vi "deviceAnalysisTest_StaticOnly.vi"() -> ()   [LabVIEW 2017]
uses:
  <vilib>/addons/InsightCM/MessageBus/Base/KeyValuePairs.ctl
  <vilib>/addons/InsightCM/MessageBus/Base/controls/AlarmRuleEntry.ctl
  <vilib>/addons/InsightCM/Devices/Shared/DataAccessors/controls/channelType_StatusLookup.ctl
  <vilib>/addons/InsightCM/MessageBus/Base/ConfigurableMetric.ctl
  <vilib>/addons/InsightCM/Utilities/ChannelStatus/controls/status.ctl
  <vilib>/addons/InsightCM/Utilities/ChannelStatus/controls/statusState.ctl
  <vilib>/addons/InsightCM/Devices/Shared/ConfigurationParsing/controls/filePaths.ctl
panel:
  out "status changed":bool
  in  "milliseconds to wait":u32=100
  in  "Tab Control":T1(tab)
  in  "Root Directory":path=path "C:/Users/Administrator/Desktop/testDevice files/speedProfile"
  in  "Configuration Files":T2={"AlarmRules"=path "AlarmRules.json", "MetricCfg"=path "MetricConfigs.json", "HierarchyNode"=path "Hierarchy.json", "DeviceModel"=path "DeviceModel.json"}
  in  "Static Values":dbl[](array[numeric])
  out "Waveform Graph":waveform(dbl)[](graph)
  out "FeatureLookup":variant
  in  "stop":bool
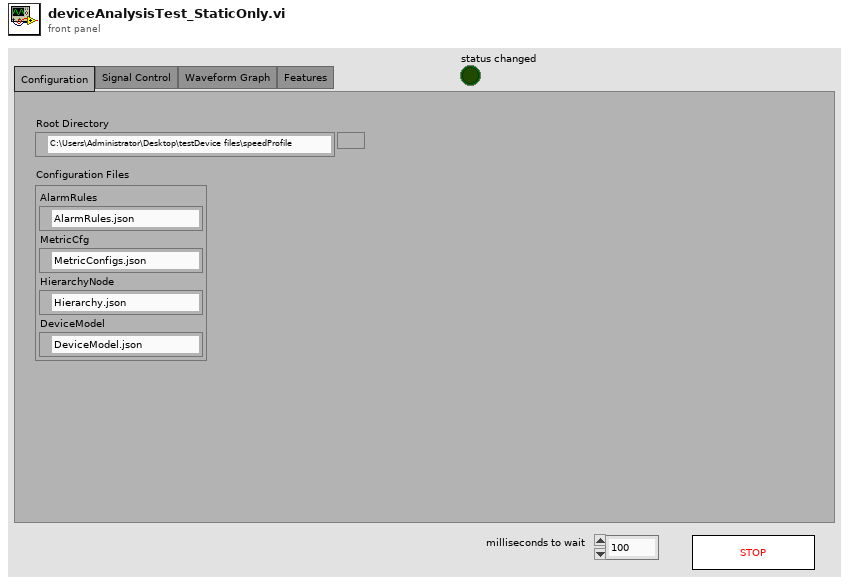
[diagram p1: front panel]
types:
  T1 = enum32{"Configuration", "Signal Control", "Waveform Graph", "Features"}
  T2 = typedef "ConfigurationParsing.lvlib/filePaths.ctl" = cluster{"AlarmRules":path, "MetricCfg":path, "HierarchyNode":path, "DeviceModel":path}
  T3 = typedef "ChannelStatus.lvlib/statusState.ctl" = cluster{"channelAlias":string, "current":T4, "previous":T4, "changed":bool}
  T4 = typedef "ChannelStatus.lvlib/status.ctl" = enum16{"init", "ok", "open", "short", "outOfRange"}
  T5 = typedef "ConfigurableMetric.ctl" = cluster{"Id":i32, "MetricType":string, "Name":string, "Locked":bool, "Properties":T6}
  T6 = typedef "KeyValuePairs.ctl" = cluster{"Key":string, "Value":string}[]
  T7 = typedef "AlarmRuleEntry.ctl" = cluster{"Id":i32, "State":string, "Path":string, "Message":string, "DeviceOnly":bool, "Configuration":cluster{"Condition":string, "SetPoint":string, "Type":string, "Hysteresis":dbl, "OnDelaySeconds":dbl, "OffDelaySeconds":dbl}, "Severity":i32}
  T8 = typedef "ConfigurationParsing.lvlib/DeviceConfigData.ctl" = cluster{"Device Info":T9, "AcquisitionProperties":variant, "Channels":variant[], "StreamingProperties":variant, "DeviceSystemProperties":variant}
  T9 = typedef "ConfigurationParsing.lvlib/deviceInfo.ctl" = cluster{"Config Version":string, "DeviceID":string}
  T10 = typedef "DeviceModel.ctl" = cluster{"AssetModel":T11, "SoftwareModel":T12}
  T11 = typedef "AssetModel.ctl" = cluster{"Id":i32, "PhysicalName":string, "LogicalName":string, "PluginCodename":string, "FirmwareInfo":string, "HardwareConfig":string, "SoftwareConfigId":i32, "HierarchyNodeId":i32}
  T12 = typedef "SoftwareModel.ctl" = cluster{"Id":i32, "DeviceAssetModelId":i32, "Version":string, "Config":string, "DeviceProperties":T6, "Channels":T13[]}
  T13 = typedef "BlueRidgeChannel.ctl" = cluster{"Id":i32, "ChannelId":string, "Name":string, "ChannelCategory":string, "ChannelType":string, "ChannelTypeList":string, "HierarchyNodeId":i32, "Enabled":bool, "Properties":T6, "MetricConfigurations":T14[]}
  T14 = typedef "MetricConfiguration.ctl" = cluster{"Id":i32, "ChannelCategory":string, "MeasurementType":string, "Metrics":T15[]}
  T15 = typedef "MetricInstance.ctl" = cluster{"Id":i32, "Codename":string, "DisplayName":string, "Unit":string, "PublishToHistorian":bool, "Unscaled":bool, "Locked":bool, "TagPath":string, "Properties":T6}
  T16 = cluster{"AlarmRules":variant, "MetricCfg":variant, "HierarchyNode":variant, "DeviceConfig":T8, "DeviceModel":T10}
  T17 = typedef "AnalysisDevice.ctl" = cluster{"Device Id":string, "Dynamic Channels":T18[], "Static Channels":T26[]}
  T18 = typedef "AnalysisDynamicChannel.ctl" = cluster{"ChannelName":string, "Sensor Type":T19, "Conversion Op":T20, "Features":T21[], "Data":waveform(sgl), "Speed":sgl, "SP Index":i32, "Properties":variant, "Data Valid":bool, "Calc Measurement Type":T25}
  T19 = typedef "AnalysisSensorType.ctl" = enum16{"Accelerometer", "Velocity", "Displacement", "Tachometer", "Tempertature ", "dynamicVoltage", "Voltage", "Current", "Microphone", "Resistance", "Digital Input", "<Unknown>"}
  T20 = typedef "AnalysisConversionOp.ctl" = enum16{"none", "singleInt", "doubleInt", "singleDiff", "doubleDiff"}
  T21 = typedef "AnalysisFeature.ctl" = cluster{"Type":i32, "Code Name":string, "Unit":string, "Display Name":string, "Value":sgl, "Start":dbl, "Stop":dbl, "Band Domain":T22, "Band Calc":T23, "Amplitude Scale":T24, "Tag Path":string}
  T22 = typedef "AnalysisBandDomain.ctl" = enum16{"Frequency", "CPM", "Orders"}
  T23 = typedef "AnalysisBandCalculation.ctl" = enum16{"Total", "Max", "Phase"}
  T24 = typedef "AnalysisBandAmplitudeScale.ctl" = enum16{"rms", "peak", "pk-pk", "phase", "<none>"}
  T25 = typedef "AnalysisCalculatedMeasurementType.ctl" = enum16{"acceleration", "velocity", "displacement", "tachometer", "speed", "temperature", "voltage", "current", "resistance", "digitalInput", "<Unknown>"}
  T26 = typedef "AnalysisStaticChannel.ctl" = cluster{"ChannelName":string, "Sensor Type":T19, "Features":T21[], "Properties":variant, "Data Valid":bool, "Calc Measurement Type":T25, "Acquisition Timestamp":timestamp}
  T27 = typedef "AnalysisState.ctl" = cluster{"Properties":cluster{"File Properties":variant, "Static Properties":variant, "Waveform Properties":variant}, "Properties Initialized?":bool, "Device":T17, "Speed Profiles":T28[]}
  T28 = typedef "AnalysisSpeedProfile.ctl" = cluster{"t0":dbl, "pulse positions":sgl[], "speed":dbl}
  T29 = typedef "AnalysisBOP.lvlib/AnalysisGroups.ctl" = cluster{"StaticChannels":T30[], "TachVibrationGroups":T32[]}
  T30 = typedef "AnalysisBOP.lvlib/GeneralStaticChanAnalysisCfg.ctl" = cluster{"Wfm Index":i32, "ChannelName":string, "ChannelID":string, "bounds":T31, "TagPath":string, "Triggerable":bool}
  T31 = typedef "ChannelStatus.lvlib/outOfRangeBounds.ctl" = cluster{"maximum":dbl, "minimum":dbl}
  T32 = typedef "AnalysisBOP.lvlib/TachVibrationGroupCfg.ctl" = cluster{"TachometerChanAnalysisConfig":T33, "AnalysisChannels":T34[]}
  T33 = typedef "AnalysisBOP.lvlib/TachometerChanAnalysisCfg.ctl" = cluster{"Wfm Index":i32, "ChannelName":string, "ChannelID":string, "PulsesPerRevolution":sgl, "TachometerThreshold":sgl, "TachometerSlope":string, "TachometerHysteresis":sgl, "sampleRate":dbl, "tachometerType":string, "Analysis Wfm Index":i32}
  T34 = typedef "AnalysisBOP.lvlib/VibrationChanAnalysisCfg.ctl" = cluster{"Wfm Index":i32, "ChannelName":string, "ChannelID":string, "speedRatio":dbl, "MeasurementType":string}
  T35 = typedef "channelType_StatusLookup.ctl" = enum16{"Static", "Dynamic"}
  T36 = typedef "wfmSGL_DVR.ctl" = refnum<data-value>
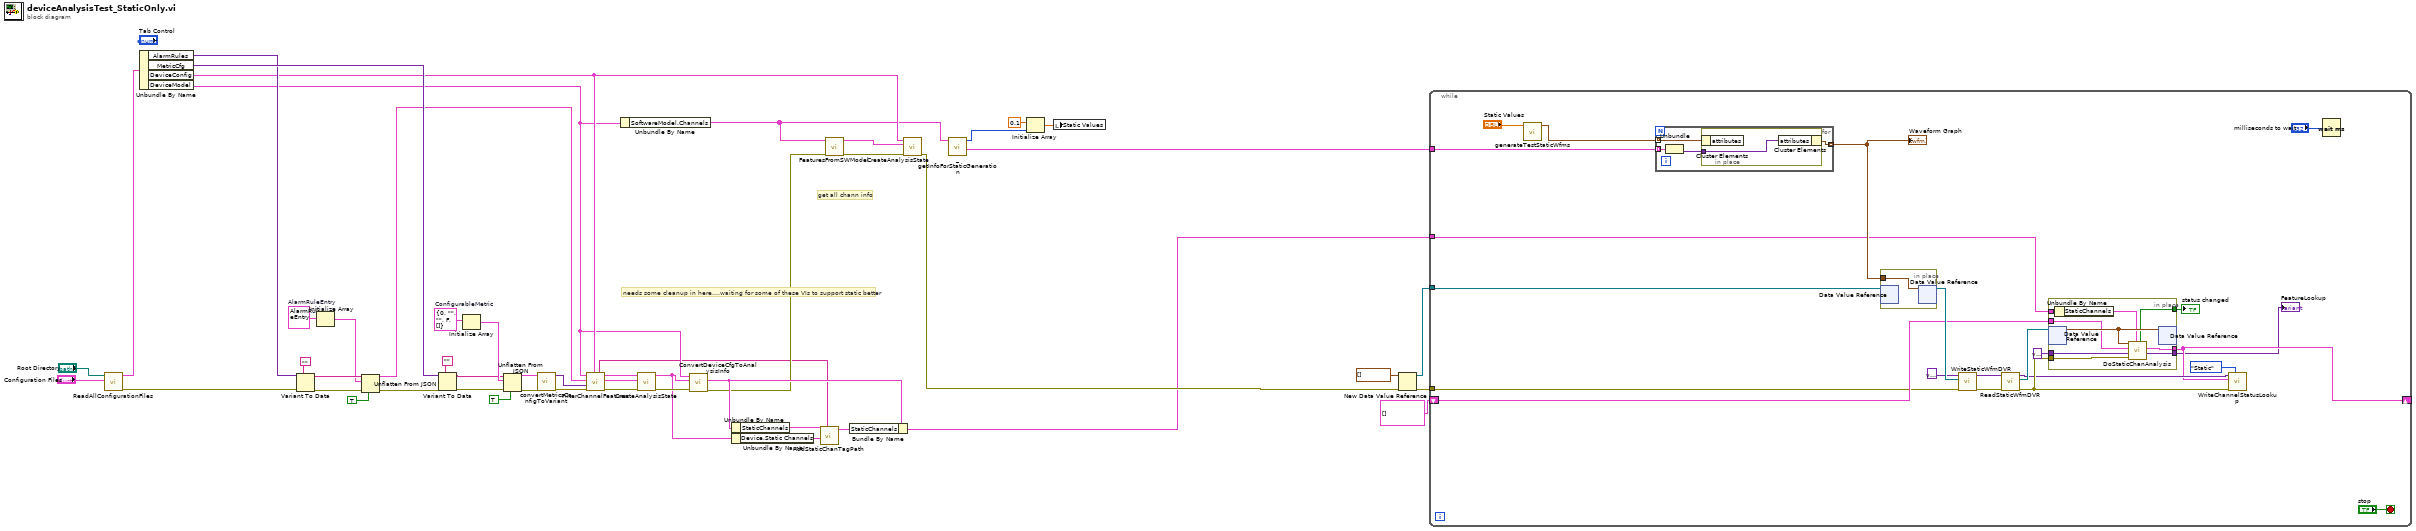
[diagram p0: block diagram]
diagram:
  w22 = T5 {"Id"=0, "MetricType"="", "Name"="", "Locked"=FALSE, "Properties"=[]}  # ConfigurableMetric
  w34 = T7 {"Id"=0, "State"="", "Path"="", "Message"="", "DeviceOnly"=FALSE, "Configuration"={"Condition"="", "SetPoint"="", "Type"="", "Hysteresis"=0.0, "OnDelaySeconds"=0.0, "OffDelaySeconds"=0.0}, "Severity"=0}  # AlarmRuleEntry
  # "needs some cleanup in here....waiting for some of these VIs to support static better"
  # "get all chann info"
  n1 = call <vilib>:"ReadAllConfigurationFiles.vi"("Configuration Files"="Configuration Files", "Root Directory"="Root Directory") -> ("error out"=w7:errorcluster, "Configuration"=w46:T16)  [unwired: 6 in, 2 out]
  n2 = Unbundle By Name(w46) -> ("AlarmRules"=w31:variant, "MetricCfg"=w40:variant, "DeviceConfig"=w20:T8, "DeviceModel"=w3:T10)
  n3 = Variant To Data(error in=w7, type="", Variant=w31) -> (data=w35:string, error out=w37:errorcluster)
  n4 = Initialize Array(w34) -> (w33:T7[])  [unwired: 1 in]
  n5 = Unflatten From JSON(JSON string=w35, type and defaults=w33, default null elements? (F)=TRUE, error in (no error)=w37) -> (value=w23:T7[], error out=w32:errorcluster)  [unwired: 3 in]
  n6 = Variant To Data(error in=w32, type="", Variant=w40) -> (data=w41:string, error out=w44:errorcluster)
  n7 = Initialize Array(w22) -> (w42:T5[])  [unwired: 1 in]
  n8 = Unflatten From JSON(JSON string=w41, type and defaults=w42, default null elements? (F)=TRUE, error in (no error)=w44) -> (value=w39:T5[], error out=w30:errorcluster)  [unwired: 3 in]
  n9 = call <vilib>:"convertMetricsConfigToVariant.vi"("error in (no error)"=w30, "MetricInstanceConfigs"=w39) -> ("error out"=w47:errorcluster, "metricInstanceConfig"=w24:variant)  [unwired: 8 in]
  n10 = call <vilib>:"FilterChannelFeatures.vi"("DeviceConfig"=w20, "error in (no error)"=w47, "Metric Lookup"=w24, "AlarmRules"=w23, "DeviceModel"=w3) -> ("error out"=w50:errorcluster, "Device"=w48:T17, "DeviceConfig Out"=w49:T8, "trigger list"=w2:string[])  [unwired: 3 in]
  n11 = Unbundle By Name(w3) -> ("SoftwareModel.Channels"=w13:T13[])
  n12 = call <vilib>:"CreateAnalysisState.vi"("error in (no error)"=w50, "Device"=w48, "DeviceConfig"=w49) -> ("error out"=w6:errorcluster, "Analysis State"=w4:T27)  [unwired: 7 in]
  n13 = call <vilib>:"ConvertDeviceCfgToAnalysisInfo.vi"("error in (no error)"=w6, "Analysis State"=w4, "DeviceModel"=w3) -> ("error out"=w5:errorcluster, "AnalysisGroups"=w9:T29)  [unwired: 5 in, 2 out]
  n14 = Unbundle By Name(w9) -> ("StaticChannels"=w11:T30[])
  n15 = Unbundle By Name(w4) -> ("Device.Static Channels"=w12:T26[])
  n16 = call <vilib>:"AddStaticChanTagPath.vi"("trigger list"=w2, "Device.Static Channels"=w12, "StaticChannels"=w11) -> ("StaticChannels out"=w10:T30[])  [unwired: 8 in]
  n17 = call <vilib>:"FeaturesFromSWModel.vi"("error in (no error)"=w5, "Channels"=w13) -> ("error out"=w15:errorcluster, "Device"=w14:T17)  [unwired: 8 in]
  n18 = Bundle By Name(cluster=w9, "StaticChannels"=w10) -> (w8:T29)
  n19 = call <vilib>:"CreateAnalysisState.vi"("error in (no error)"=w15, "Device"=w14, "DeviceConfig"=w20) -> ("error out"=w21:errorcluster)  [unwired: 7 in, 1 out]
  n20 = call <vilib>:"_getInfoForStaticGeneration.vi"("Channels"=w13) -> ("wfm info"=w19:cluster{i32, "variant":variant}[], "number of channels"=w18:i32)  [unwired: 9 in]
  n21 = Initialize Array(0.1 ("element"), w18) -> (w16:dbl[])
  n22 = local write "Static Values"(w16) -> ()
  n23 = New Data Value Reference(data value=waveform(sgl)[] [] ("wfmData"), error in=w21) -> (data value reference=w26:refnum<data-value>, error out=w27:errorcluster)
  n24 = while {
    tunnel: w27 -> [w53]
    tunnel: w8 -> [w54]
    shift-right: [w59] -> _
    shift-left: T3[] [] ("channel status") -> [w57]
    tunnel: w26 -> [w72]
    tunnel: w19 -> [w68]
    stop <- "stop" stop-if-true
    n25 = call <vilib>:"generateTestStaticWfms.vi"("Static Values"="Static Values") -> ("waveforms"=w52:waveform(dbl)[])  [unwired: 10 in]
    n26 = for {
      tunnel: w52 -> [w84] mode=indexing
      tunnel: w68 -> [w85] mode=indexing
      tunnel: [w83] -> w67 mode=indexing
      n27 = Unbundle(w85) -> ("variant"=w82:variant)  [unwired: 1 out]
      n28 = in-place {
        in-place-border: w82 -> [w86]
        n29 = in-place-cluster #1(w84) -> ()  [unwired: 1 out]
        n30 = in-place-cluster #1("attributes"=w86) -> (w83:waveform(dbl))
      }
    }
    "Waveform Graph" <- w67
    n31 = in-place {
      in-place-border: w67 -> [w87]
      n32 = in-place-dvr #2(w72) -> ()  [unwired: 2 out]
      n33 = in-place-dvr #2(w87) -> (w71:refnum<data-value>)  [unwired: 1 out]
    }
    n34 = call <vilib>:"WriteStaticWfmDVR.vi"("error in (no error)"=w53, "staticWfmDVR"=w71, "variant"=variant) -> ("error out"=w61:errorcluster, "variant"=w60:variant)  [unwired: 7 in]
    n35 = call <vilib>:"ReadStaticWfmDVR.vi"("error in (no error)"=w61, "variant"=w60) -> ("error out"=w63:errorcluster, "staticWfmDVR"=w66:T36, "variant"=w62:variant)  [unwired: 7 in]
    n36 = in-place {
      in-place-border: w63 -> [w81]
      in-place-border: variant ("variant") -> [w78]
      in-place-border: [w80] -> w56
      in-place-border: [w77] -> w59
      in-place-border: [w76] -> w55
      in-place-border: w57 -> [w75]
      in-place-border: w54 -> [w73]
      n37 = in-place-dvr #3(w66) -> (w79:waveform(sgl)[])  [unwired: 1 out]
      n38 = Unbundle By Name(w73) -> ("StaticChannels"=w74:T30[])
      n39 = call <vilib>:"DoStaticChanAnalysis.vi"("StaticChannels"=w74, "error in (no error)"=w81, "FeatureLookup"=w78, "channel status"=w75, "waveforms"=w79) -> ("FeatureLookup"=w80:variant, "channel status"=w77:T3[], "status changed"=w76:bool)  [unwired: 2 in, 2 out]
      n40 = in-place-dvr #3(w79) -> ()  [unwired: 2 out]
    }
    "FeatureLookup" <- w56
    "status changed" <- w55
    n41 = call <vilib>:"WriteChannelStatusLookup.vi"("channel type"=channelType_StatusLookup."Static", "error in (no error)"=w63, "channel status"=w59, "variant"=w62) -> ()  [unwired: 6 in, 2 out]
    n42 = Wait (ms)(milliseconds to wait="milliseconds to wait") -> ()  [unwired: 1 out]
  }
